vi "Succeed.vi"(7 "Name":string="Succeed", 11 "Node In":refnum<class "abs_Node.lvclass">) -> (3 "Node":refnum<class "abs_Node.lvclass">)   [LabVIEW 2021, in "BT.lvlib"]
uses:
  BT.lvlib
  Succeed/Succeed.lvclass
  C:/Users/Tim/Documents/LabVIEW/2021/Behaviour Tree/abs_Node/abs_Node.lvclass
  abs_Node/abs_Node.lvclass
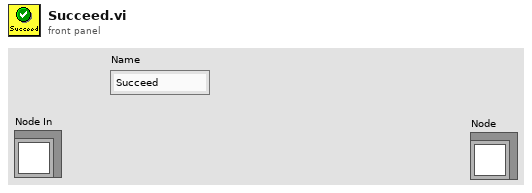
[diagram p1: front panel]
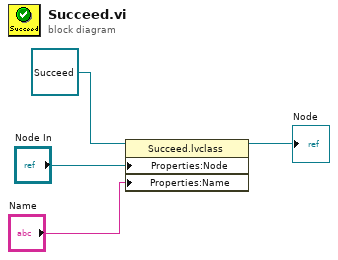
[diagram p0: block diagram]
diagram:
  n1 = property class="Succeed.lvclass"(reference=refnum<class "Succeed.lvclass"> refnum ("BT.lvlib:Succeed.lvclass"), "Properties:Node"="Node In", "Properties:Name"="Name") -> (reference out=→"Node":refnum<class "Succeed.lvclass">)  [unwired: 1 in, 1 out]
